vi "interpolate.issue.dates.vi"(9 "dup issues":i32[](array[numeric]), 11 "issues":T1[](array[typedef]) {"display_date" format="%<%x>T"}) -> (3 "issues out":T1[](array[typedef]) {"display_date" format="%<%x>T"})   [LabVIEW 2024]
uses:
  CV_RESTful_Library/typedefs/local_issue--cluster.ctl
  CV_RESTful_Library/typedefs/cv_issue.generic_credit--cluster.ctl
  CV_RESTful_Library/typedefs/cv_issue.associated_image--cluster.ctl
  CV_RESTful_Library/typedefs/cv_issue.person_credit--cluster.ctl
  CV_RESTful_Library/CV_RESTful_Lib.lvlib
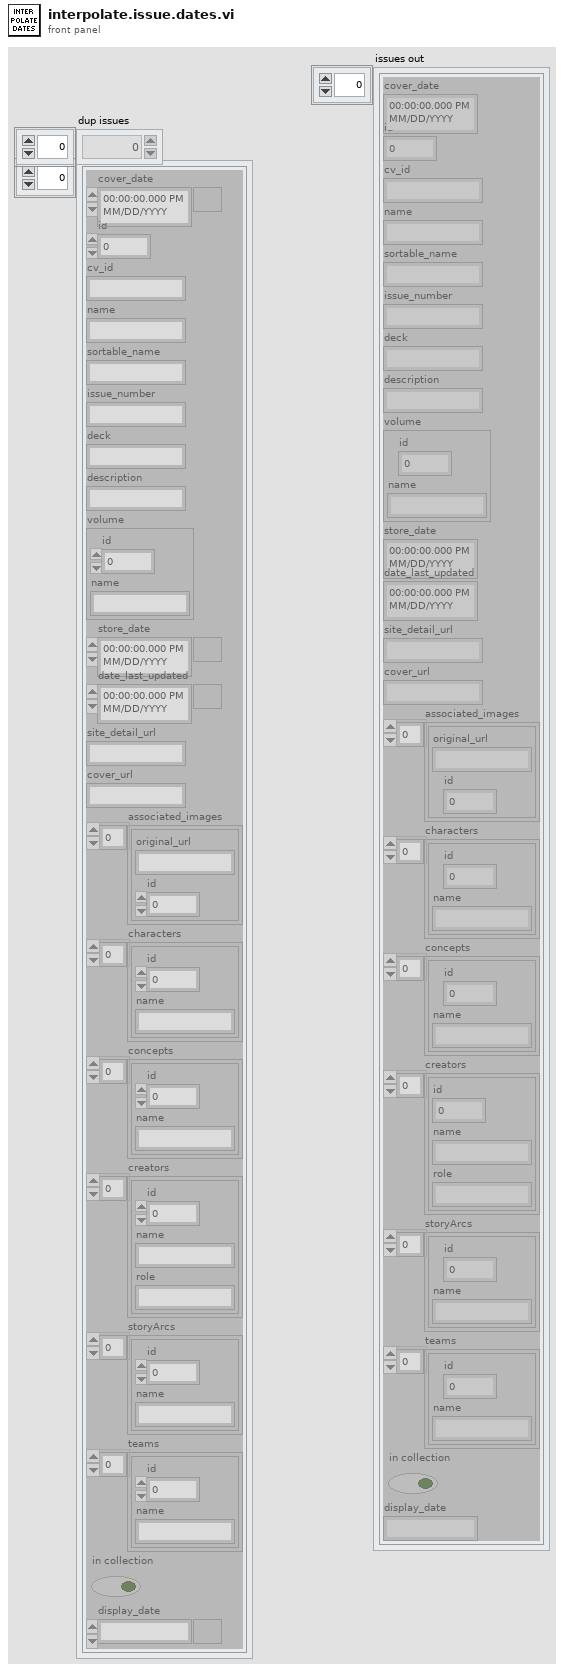
[diagram p1: front panel]
types:
  T1 = typedef "CV_RESTful_Lib.lvlib/local_issue--cluster.ctl" = cluster{"cover_date":timestamp, "id":i32, "cv_id":string, "name":string, "sortable_name":string, "issue_number":string, "deck":string, "description":string, "volume":T2, "store_date":timestamp, "date_last_updated":timestamp, "site_detail_url":string, "cover_url":string, "associated_images":T3[], "characters":T2[], "concepts":T2[], "creators":T4[], "storyArcs":T2[], "teams":T2[], "in collection":bool, "display_date":timestamp}
  T2 = typedef "CV_RESTful_Lib.lvlib/cv_issue.generic_credit--cluster.ctl" = cluster{"id":i32, "name":string}
  T3 = typedef "CV_RESTful_Lib.lvlib/cv_issue.associated_image--cluster.ctl" = cluster{"original_url":string, "id":i32}
  T4 = typedef "CV_RESTful_Lib.lvlib/cv_issue.person_credit--cluster.ctl" = cluster{"id":i32, "name":string, "role":string}
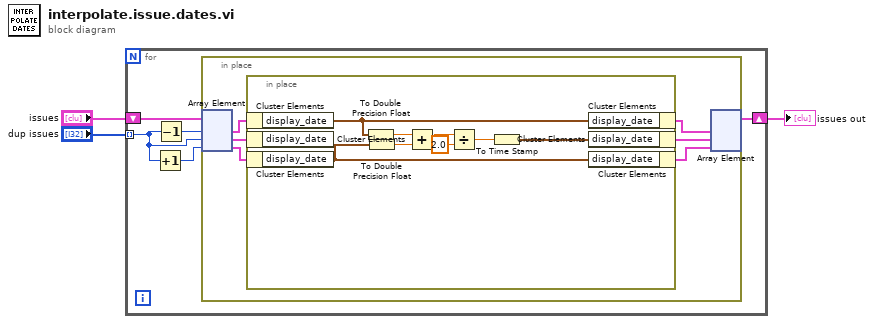
[diagram p0: block diagram]
diagram:
  n1 = for {
    tunnel: "dup issues" -> [w4] mode=indexing
    shift-right: [w7] -> w1
    shift-left: "issues" -> [w8]
    n2 = Increment(x=w4) -> (x+1=w6:i32)
    n3 = Decrement(x=w4) -> (x-1=w5:i32)
    n4 = in-place {
      n5 = in-place-array #1(w8, w5, w4, w6) -> (w14:T1, w13:T1, w12:T1)
      n6 = in-place {
        n7 = in-place-cluster #2(w14) -> ("display_date"=w15:timestamp)
        n8 = in-place-cluster #3(w13) -> ()  [unwired: 1 out]
        n9 = in-place-cluster #4(w12) -> ("display_date"=w16:timestamp)
        n10 = To Double Precision Float(number=w15) -> (double precision float=w22:dbl)
        n11 = To Double Precision Float(number=w16) -> (double precision float=w21:dbl)
        n12 = Add(x=w22, y=w21) -> (x+y=w20:dbl)
        n13 = Divide(x=w20, y=2.0) -> (x/y=w18:dbl)
        n14 = To Time Stamp(1:w18) -> (0:w17:timestamp)
        n15 = in-place-cluster #2("display_date"=w15) -> (w11:T1)
        n16 = in-place-cluster #3("display_date"=w17) -> (w9:T1)
        n17 = in-place-cluster #4("display_date"=w16) -> (w10:T1)
      }
      n18 = in-place-array #1(w11, w9, w10) -> (w7:T1[])  [unwired: 3 out]
    }
  }
  "issues out" <- w1
